vi "PQsendDescribePrepared.vi"(8 "error in (no error)":errorcluster, 10 "stmt":string, 11 "conn":u32) -> (0 "error out":errorcluster, 2 "PQsendQueryPrepared":u32, 3 "conn_out":u32)   [LabVIEW 2019, in "libpqlv.lvlib"]
uses:
  libpqlv.lvlib
  libpq.dll
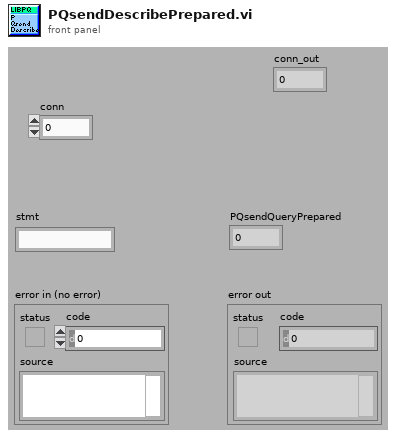
[diagram p1: front panel]
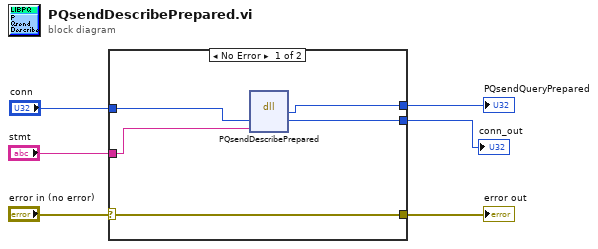
[diagram p0: block diagram]
diagram:
  n1 = case shown="No Error" "error in (no error)" {
    selector: "error in (no error)" -> [w11 w13]
    tunnel: [w11 w13] -> w5
    tunnel: [w10 _] -> w4
    tunnel: "stmt" -> [w9 _]
    tunnel: "conn" -> [w8 w12]
    tunnel: [w7 w12] -> w1
    frame No Error {
      n2 = dll-call lib="libpq.*" fn="PQsendDescribePrepared"("conn"=w8, "stmt"=w9) -> ("PQsendDescribePrepared"=w10:u32, "conn"=w7:u32)  [unwired: 4 in, 2 out]
    }
    frame Error {
    }
  }
  "PQsendQueryPrepared" <- w4
  "error out" <- w5
  "conn_out" <- w1
